vi "Pause.vi"(8 "error in (no error)":errorcluster, 10 "Internal?":bool, 11 "Huber Settings":T1) -> (0 "error out":errorcluster, 3 "Huber Settings":T1)   [LabVIEW 2018, in "Lauda TCU.lvlib"]
uses:
  Lauda TCU.lvlib
  Lauda Settings.ctl
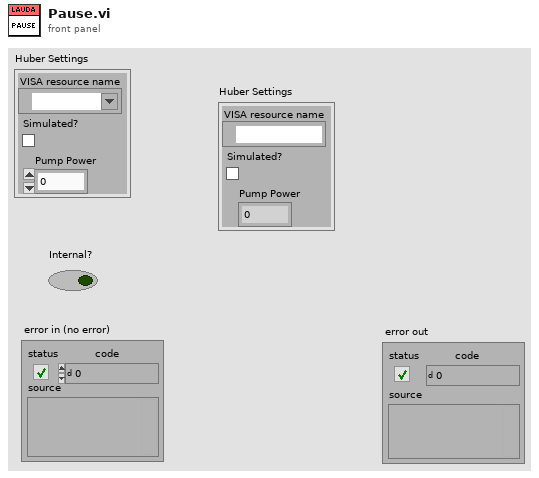
[diagram p1: front panel]
types:
  T1 = typedef "Lauda TCU.lvlib/Lauda Settings.ctl" = cluster{"VISA resource name":refnum<visa-resource-name>, "Simulated?":bool, "Pump Power":i32}
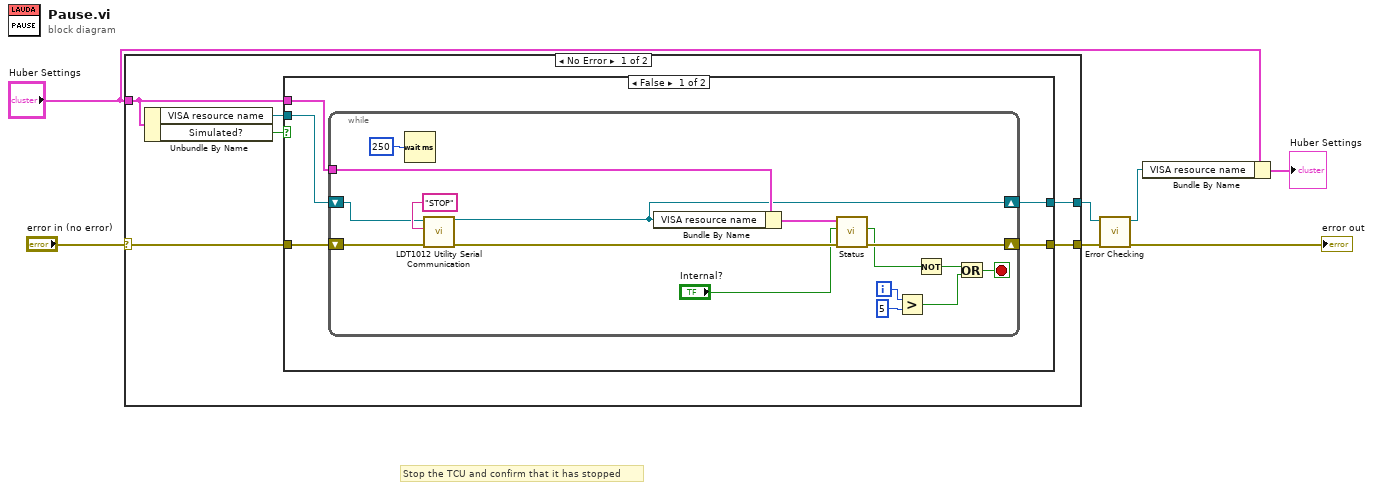
[diagram p0: block diagram]
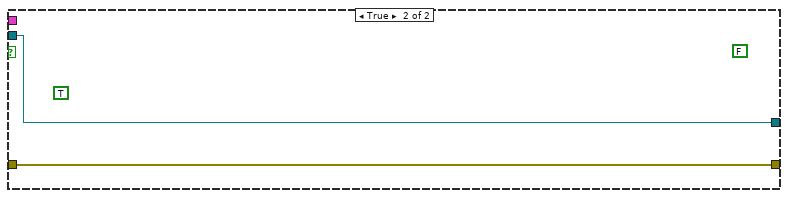
[diagram p2: hidden frame]
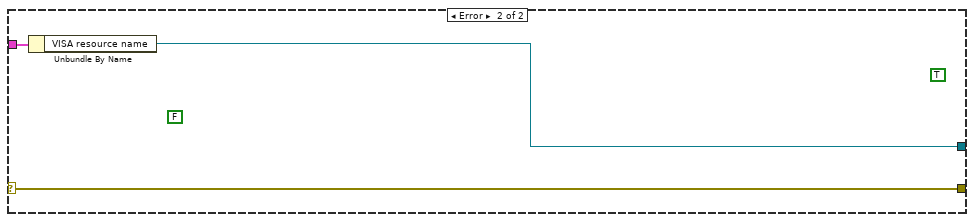
[diagram p3: hidden frame]
diagram:
  # "Stop the TCU and confirm that it has stopped"
  n1 = case shown="No Error" "error in (no error)" {
    selector: "error in (no error)" -> [w13 w39]
    tunnel: "Huber Settings" -> [w8 w38]
    tunnel: [w12 w39] -> w5
    tunnel: [w10 w37] -> w6
    frame No Error {
      n2 = Unbundle By Name(w8) -> ("VISA resource name"=w11:refnum<visa-resource-name>, "Simulated?"=w9:bool)
      n3 = case shown="False" w9 {
        tunnel: w13 -> [w16 w36]
        tunnel: [w14 w36] -> w12
        tunnel: [w18 w35] -> w10
        tunnel: w11 -> [w17 w35]
        tunnel: w8 -> [w15 _]
        frame False {
          n4 = while {
            tunnel: w15 -> [w22]
            shift-right: [w20] -> w18
            shift-left: w17 -> [w24]
            shift-right: [w34] -> w14
            shift-left: w16 -> [w23]
            i -> [w32]
            stop <- w33 stop-if-true
            n5 = Wait (ms)(milliseconds to wait=u32 250) -> ()  [unwired: 1 out]
            n6 = call "LDT1012 Utility Serial Communication.vi"("error in (no error)"=w23, "Command String"="STOP", "VISA session"=w24) -> ("error out"=w25:errorcluster, "dup VISA session"=w20:refnum<visa-resource-name>)  [unwired: 5 in, 2 out]
            n7 = Bundle By Name(cluster=w22, "VISA resource name"=w20) -> (w21:T1)
            n8 = call "Status.vi"("error in (no error)"=w25, "Internal?"="Internal?", "Lauda Settings"=w21) -> ("error out"=w34:errorcluster, "Running"=w28:bool)  [unwired: 2 in, 5 out]
            n9 = Greater?(x=w32, y=5) -> (0:w30:bool)
            n10 = Not(x=w28) -> (.not. x?=w27:bool)
            n11 = Or(x=w27, y=w30) -> (x .or. y?=w33:bool)
          }
        }
        frame True {
          (unwired) TRUE
          (unwired) FALSE
        }
      }
    }
    frame Error {
      (unwired) FALSE
      (unwired) TRUE
      n12 = Unbundle By Name(w38) -> ("VISA resource name"=w37:refnum<visa-resource-name>)
    }
  }
  n13 = call "Error Checking.vi"("error in (no error)"=w5, "VISA resource name"=w6) -> ("error out"=→"error out":errorcluster, "VISA resource name"=w3:refnum<visa-resource-name>)  [unwired: 7 in, 1 out]
  n14 = Bundle By Name(cluster="Huber Settings", "VISA resource name"=w3) -> (→"Huber Settings":T1)
